vi "HTRB Config.vi"(7 "IN Config":T1 {"Vdss Setting"."1 Step Time" format="%.1f S"; "Vdss Setting"."Step" format="%.d Step"; "Vdss Setting"."Operating Voltage [Vdss]" format="%.d V"; "Group Setting"."G3. Current Limit" format="%.2f mA"; "Group Setting"."G2. Current Limit" format="%.2f mA"; "Group Setting"."G1. Current Limit" format="%.2f mA"}, 8 "error in (no error)":errorcluster caption="에러 입력(에러 없음)") -> (0 "error out":errorcluster caption="에러 출력", 3 "OUT Config":T1 {"Vdss Setting"."1 Step Time" format="%.1f S"; "Vdss Setting"."Step" format="%.d Step"; "Vdss Setting"."Operating Voltage [Vdss]" format="%.d V"; "Group Setting"."G3. Current Limit" format="%.2f mA"; "Group Setting"."G2. Current Limit" format="%.2f mA"; "Group Setting"."G1. Current Limit" format="%.2f mA"})   [LabVIEW 2017]
uses:
  Controls/(Ctrl) Config.ctl
  <vilib>/Utility/miscctls.llb/LVPointTypeDef.ctl
  <vilib>/Utility/xml.llb/Write to XML File(string).vi
  <vilib>/Utility/xml.llb/Read From XML File(string).vi
panel:
  in  "Config":T1={"Group Setting"={"Test Group"={"Group 1"=FALSE, "Group 2"=FALSE, "Group 3"=FALSE}, "G1. Current Limit"=0.0, "G2. Current Limit"=0.0, "G3. Current Limit"=0.0}, "Vdss Setting"={"Operating Voltage [Vdss]"=1000.0, "Step"=10.0, "1 Step Time"=1.0}, "Save"={"Data Save Path"=path ""}} {"Vdss Setting"."1 Step Time" format="%.1f S"; "Vdss Setting"."Step" format="%.d Step"; "Vdss Setting"."Operating Voltage [Vdss]" format="%.d V"; "Group Setting"."G3. Current Limit" format="%.2f mA"; "Group Setting"."G2. Current Limit" format="%.2f mA"; "Group Setting"."G1. Current Limit" format="%.2f mA"}
  in  "Close":bool
  in  "Apply":bool
  in  "Load":bool
  in  "Save":bool
  out "Init":bool
  # "설정"
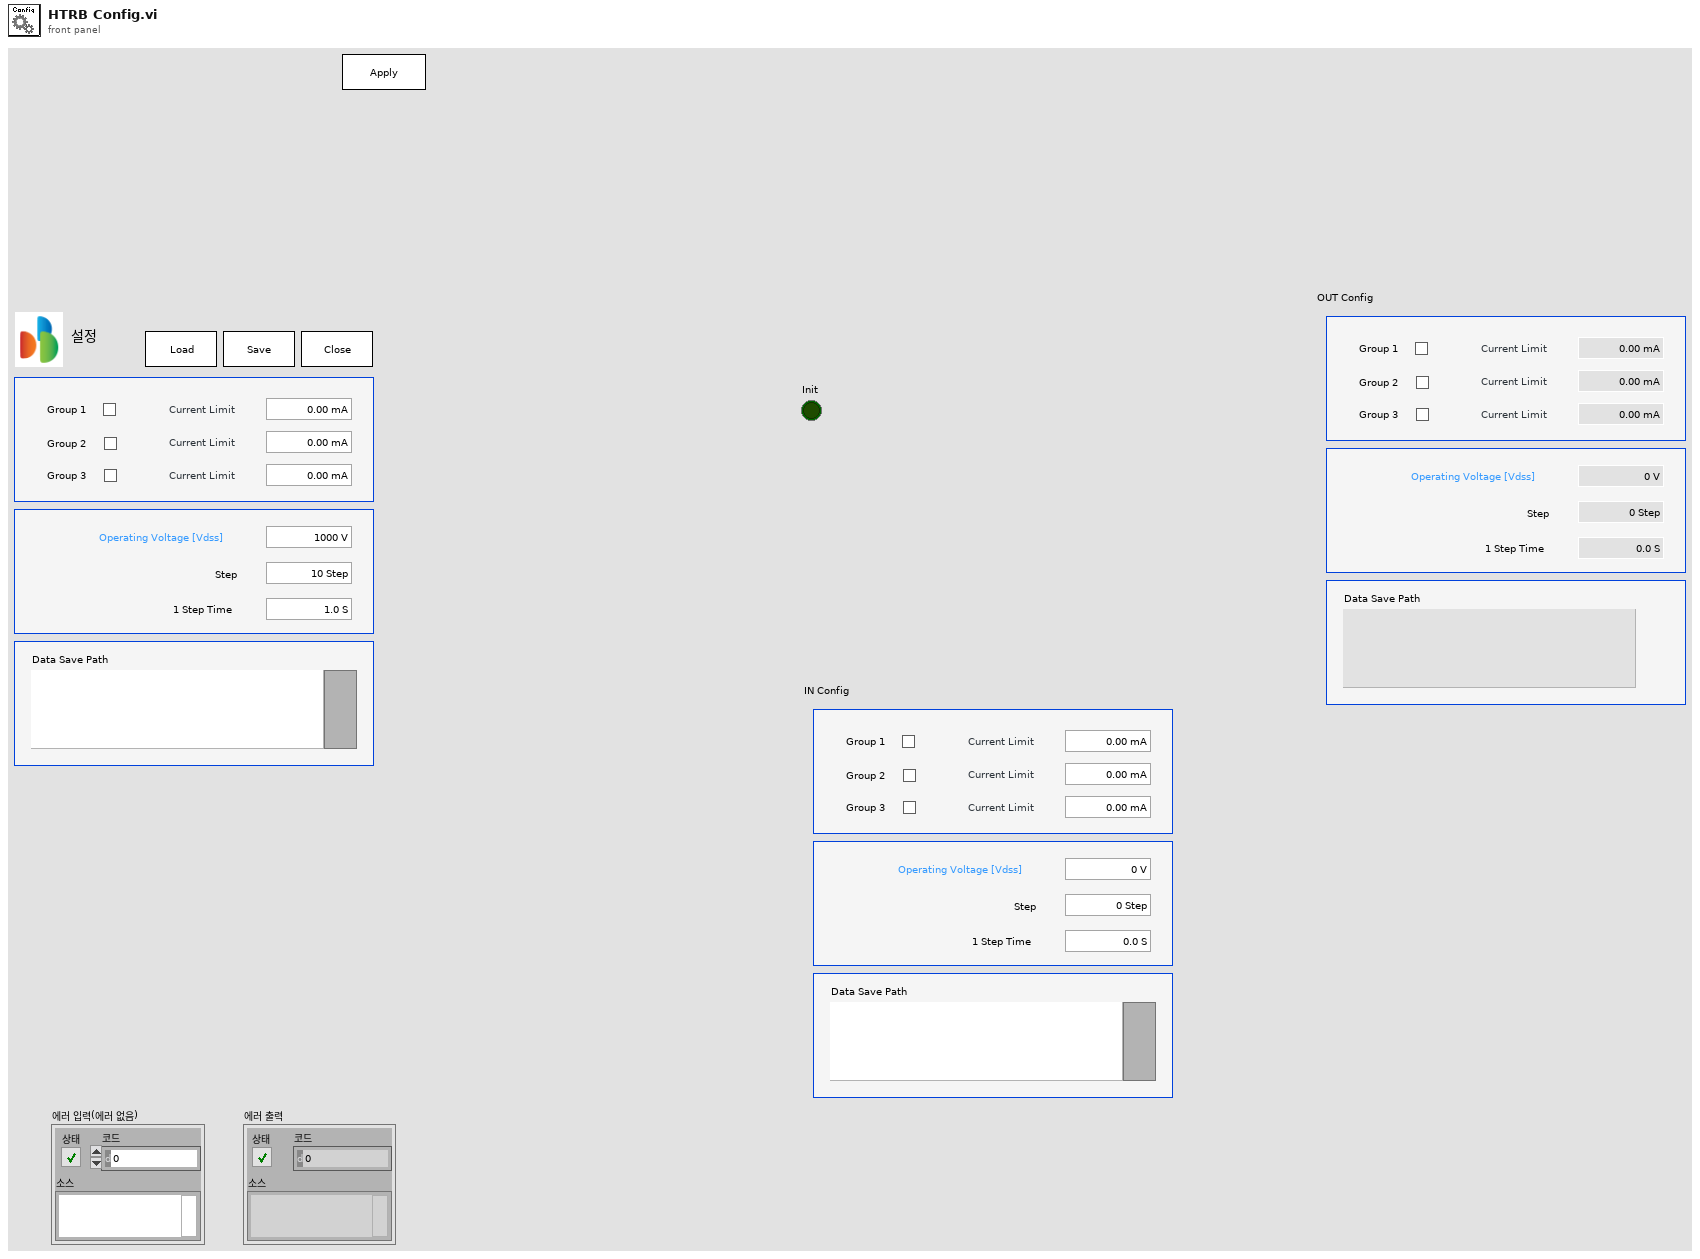
[diagram p1: front panel]
types:
  T1 = typedef "(Ctrl) Config.ctl" = cluster{"Group Setting":cluster{"Test Group":cluster{"Group 1":bool, "Group 2":bool, "Group 3":bool}, "G1. Current Limit":dbl, "G2. Current Limit":dbl, "G3. Current Limit":dbl}, "Vdss Setting":cluster{"Operating Voltage [Vdss]":dbl, "Step":dbl, "1 Step Time":dbl}, "Save":cluster{"Data Save Path":path}}
  T2 = typedef "LVPointTypeDef.ctl" = cluster{"Horizontal":i16, "Vertical":i16}
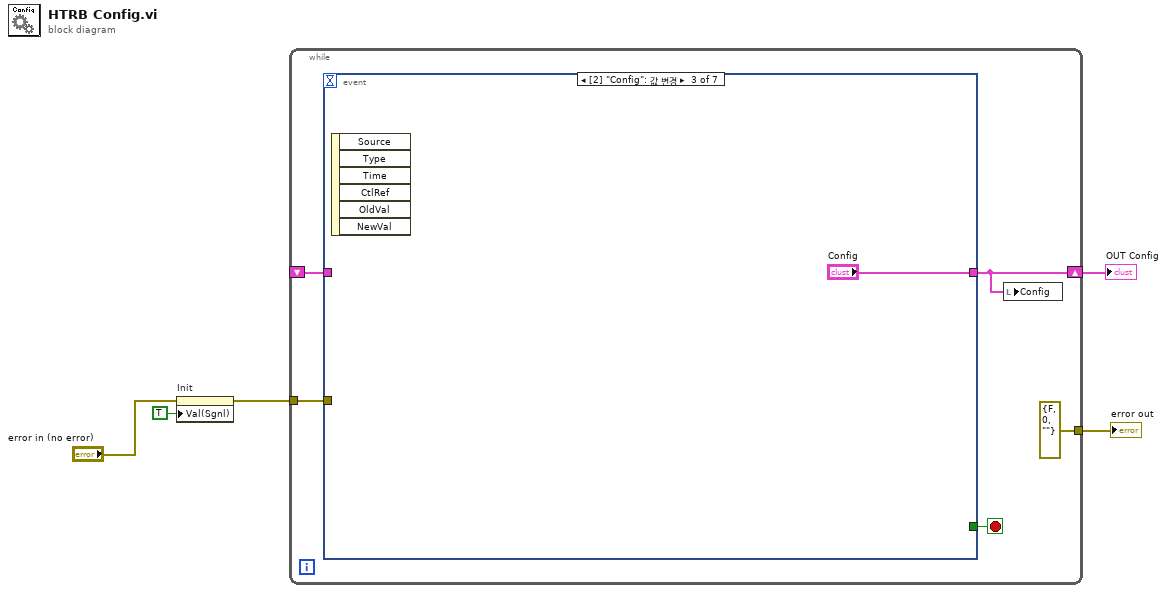
[diagram p0: block diagram]
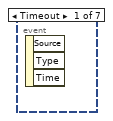
[diagram p2: hidden frame]
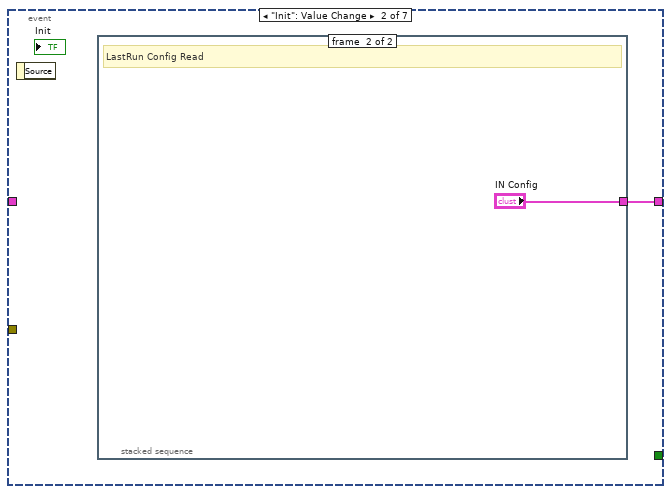
[diagram p3: hidden frame]
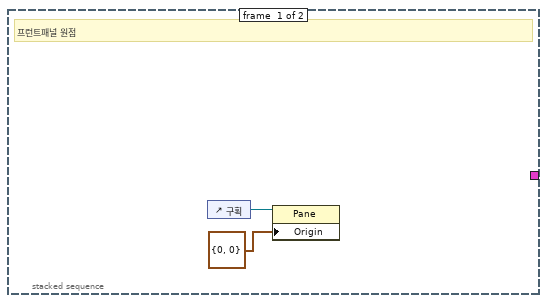
[diagram p4: hidden frame]
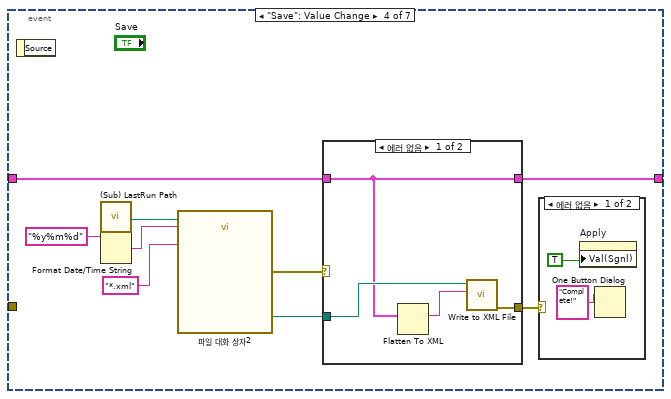
[diagram p5: hidden frame]
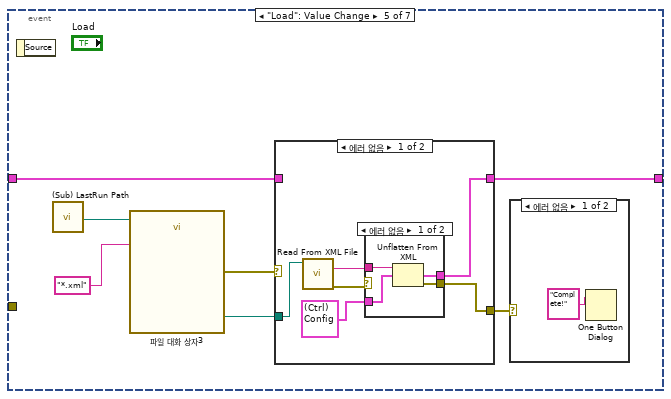
[diagram p8: hidden frame]
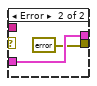
[diagram p10: hidden frame]
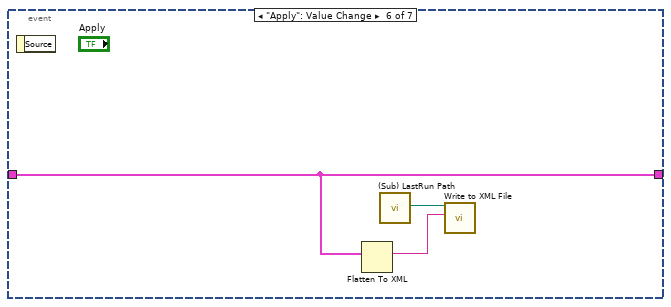
[diagram p12: hidden frame]
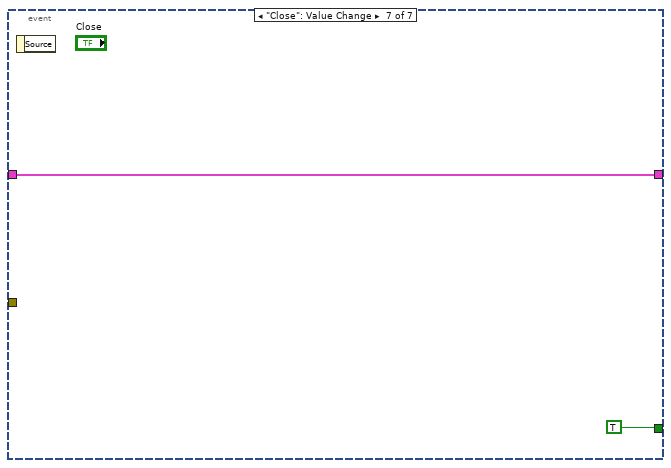
[diagram p13: hidden frame]
diagram:
  n1 = property on="Init" class="Bool (엄격한)"(error in="error in (no error)", "Val(Sgnl)"=TRUE ("값(신호)")) -> (error out=w4:errorcluster)  [unwired: 1 in, 1 out]
  n2 = while {
    tunnel: w4 -> [w6]
    shift-right: [w8] -> w1
    shift-left: _ -> [w9]
    tunnel: [errorcluster {"status"=FALSE, "code"=0, "source"=""} ("에러 상수")] -> w2
    stop <- w10 stop-if-true
    n3 = event shown="[2] \"Config\": 값 변경" {
      selector: _ -> [_ _ _ _ _ _ _]
      dyn-events: _ -> [_ _ _ _ _ _ _]
      timeout: _ -> [_ _ _ _ _ _ _]
      tunnel: [_ _ _ _ _ _ TRUE] -> w10
      tunnel: [_ w11 "Config" w17 w34 w57 w58] -> w8
      tunnel: w9 -> [_ _ _ w19 w36 w57 w58]
      tunnel: w6 -> [_ _ _ _ _ _ _]
      event Timeout {
        n4 = event-data() -> ()  [unwired: 1 in, 3 out]
      }
      event "Init": Value Change {
        n5 = event-data() -> ()  [unwired: 1 in, 1 out]
        n6 = stacked-sequence {
          tunnel: [_ "IN Config"] -> w11
          frame #0 {
            # "프런트패널 원점"
            n7 = control-ref of="구획"() -> (w13:refnum<vi>)
            n8 = property class="Pane"(reference=w13, "Origin"=T2 {"Horizontal"=0, "Vertical"=0} ("원점")) -> ()  [unwired: 1 in, 2 out]
          }
          frame #1 {
            # "LastRun Config Read"
          }
        }
      }
      event Value Change {
        n9 = event-data() -> ()  [unwired: 1 in, 6 out]
      }
      event "Save": Value Change {
        n10 = event-data() -> ()  [unwired: 1 in, 1 out]
        n11 = call "(Sub) LastRun Path.vi"() -> ("Config Path"=w24:path)  [unwired: 18 in, 1 out]
        n12 = Format Date/Time String(time format string (%c)="%y%m%d" ("시간 포맷 문자열 (%c)")) -> (date/time string=w21:string)  [unwired: 2 in]
        n13 = call "파일 대화 상자2"("start path"=w24, "default name"=w21, "pattern (all files)"="*.xml") -> ("selected path"=w18:path, "error out"=w20:errorcluster)  [unwired: 9 in, 2 out]
        n14 = case shown="에러 없음" w20 {
          selector: w20 -> [_ w31]
          tunnel: w19 -> [w28 w32]
          tunnel: w18 -> [w29 _]
          tunnel: [w28 w32] -> w17
          tunnel: [w27 w31] -> w16
          frame No Error {
            n15 = Flatten To XML(anything=w28) -> (xml string=w30:string)
            n16 = call-poly <vilib>:"Write to XML File.vi"("XML Input"=w30, "XML File Path"=w29) -> ("error out"=w27:errorcluster)  [unwired: 7 in, 2 out]
          }
          frame Error {
          }
        }
        n17 = case shown="에러 없음" w16 {
          frame No Error {
            n18 = property on="Apply" class="Bool (엄격한)"("Val(Sgnl)"=TRUE ("값(신호)")) -> ()  [unwired: 2 in, 2 out]
            n19 = One Button Dialog(message="Complete!" ("메시지")) -> ()  [unwired: 1 in, 1 out]
          }
          frame Error {
          }
        }
      }
      event "Load": Value Change {
        n20 = event-data() -> ()  [unwired: 1 in, 1 out]
        n21 = call "(Sub) LastRun Path.vi"() -> ("Config Path"=w39:path)  [unwired: 18 in, 1 out]
        n22 = call "파일 대화 상자3"("start path"=w39, "pattern (all files)"="*.xml") -> ("selected path"=w35:path, "error out"=w37:errorcluster)  [unwired: 10 in, 2 out]
        n23 = case shown="에러 없음" w37 {
          selector: w37 -> [_ w53]
          tunnel: w36 -> [_ w54]
          tunnel: w35 -> [w43 _]
          tunnel: [w42 w54] -> w34
          tunnel: [w41 w53] -> w33
          frame No Error {
            n24 = call-poly <vilib>:"Read From XML File.vi"("XML File Path"=w43) -> ("error out"=w45:errorcluster, "XML Elements"=w46:string)  [unwired: 8 in, 1 out]
            n25 = case shown="에러 없음" w45 {
              tunnel: w46 -> [w50 _]
              tunnel: T1 {"Group Setting"={"Test Group"={"Group 1"=FALSE, "Group 2"=FALSE, "Group 3"=FALSE}, "G1. Current Limit"=0.0, "G2. Current Limit"=0.0, "G3. Current Limit"=0.0}, "Vdss Setting"={"Operating Voltage [Vdss]"=0.0, "Step"=0.0, "1 Step Time"=0.0}, "Save"={"Data Save Path"=path ""}} ("Config") -> [w49 w52]
              tunnel: [w48 errorcluster {"status"=FALSE, "code"=0, "source"=""} ("에러 상수")] -> w41
              tunnel: [w47 w52] -> w42
              frame No Error {
                n26 = Unflatten From XML(xml string=w50, type=w49) -> (value=w47:T1, error out=w48:errorcluster)  [unwired: 1 in]
              }
              frame Error {
              }
            }
          }
          frame Error {
          }
        }
        n27 = case shown="에러 없음" w33 {
          frame No Error {
            n28 = One Button Dialog(message="Complete!" ("메시지")) -> ()  [unwired: 1 in, 1 out]
          }
          frame Error {
          }
        }
      }
      event "Apply": Value Change {
        n29 = event-data() -> ()  [unwired: 1 in, 1 out]
        n30 = Flatten To XML(anything=w57) -> (xml string=w56:string)
        n31 = call "(Sub) LastRun Path.vi"() -> ("LastRun Path"=w55:path)  [unwired: 18 in, 1 out]
        n32 = call-poly <vilib>:"Write to XML File.vi"("XML Input"=w56, "XML File Path"=w55) -> ()  [unwired: 7 in, 3 out]
      }
      event "Close": Value Change {
        n33 = event-data() -> ()  [unwired: 1 in, 1 out]
      }
    }
    n34 = local write "Config"(w8) -> ()
  }
  "error out" <- w2
  "OUT Config" <- w1
